vi "Pressure_Multiplexer_Server3.vi"(8 "Time per Block (s)":dbl=100.0 format="%_4f", 11 "Setup filename":string) -> (0 "DAQ Error":errorcluster, 2 "Av Sampling Rate":dbl[](array[numeric]), 3 "Time Trace":T1[](array[typedef]))   [LabVIEW 2021]
uses:
  Controls/Time_Trace_Cluster.ctl
  Controls/Setup.ctl
  Controls/Save_Data.ctl
  Camera Server/Camera enum/Camera resolution.ctl
  Globals/Meas_global.vi
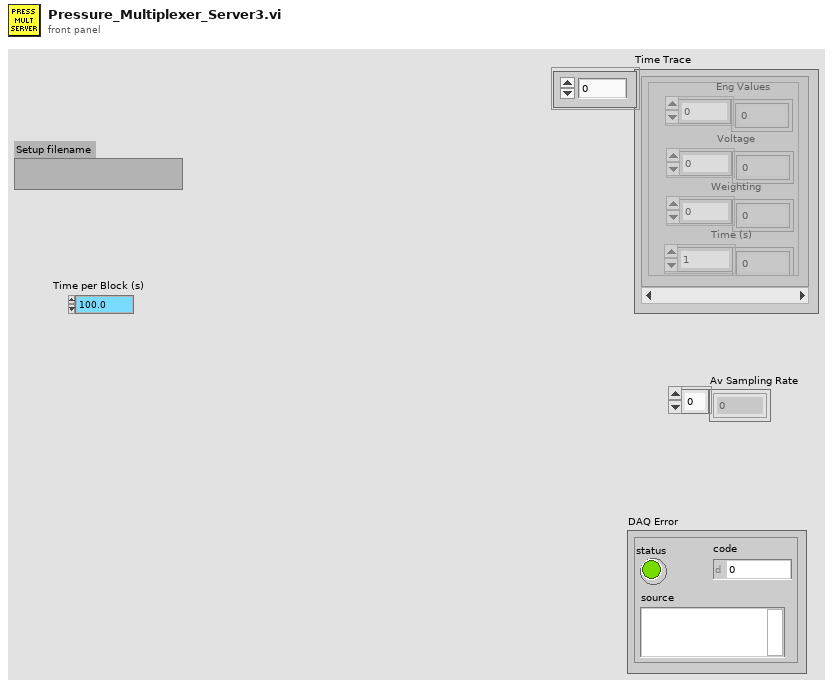
[diagram p1: front panel]
types:
  T1 = typedef "Time_Trace_Cluster.ctl" = cluster{"Weighting":dbl[], "Time (s)":dbl[], "Voltage":dbl[], "Eng Values":dbl[]}
  T2 = typedef "Save_Data.ctl" = enum16{"Save No Data", "Save Data"}
  T3 = typedef "Setup.ctl" = enum16{"Run Program", "Show Setup", "Save Current Setup", "Setup Front Panel"}
  T4 = typedef "Camera resolution.ctl" = u8
  T5 = typedef "Analysis_info_cluster.ctl" = cluster{"Colour":u32, "Inst type":T6, "Inst name":string, "Symbol":string, "Code name":string, "Extra Info":string, "Inst Array":T7, "Extra Titles":string[], "Extra Values":string[], "U":dbl, "u^2":dbl, "u^3":dbl, "u^4":dbl, "Skew_u":dbl, "Kurt_u":dbl, "Sd Error in Mean":dbl, "% u'/U":dbl, "X":dbl, "Y":dbl, "Z":dbl, "Timescale integral Estimate":dbl, "Sd Error in Variance":dbl, "Calib File":path, "Calib Constants":dbl[], "Output Position":bool, "Stats":enum16{"None", "Basic", "Full"}, "Av Sampling Rate":dbl, "Av No of Samples":dbl, "Total Meas Time (s)":dbl, "ADAM Ch Name":string, "Max value":dbl, "Min value":dbl, "Req Sample Rate Hz":dbl, "Sync Delay Time (s)":dbl, "Ch No":i16, "Device":string, "Use Latest Calib":bool, "Port":string, "Metadata Ch Names":string[], "Metadata Ch Values":string[], "Label":string}
  T6 = typedef "Inst_type.ctl" = enum16{"Raw voltage", "Raw with zero offsetting", "Propeller anemometer", "Pressure Transducer", "Pitot-static tube", "Hot wire", "Cross wire 1", "Cross wire 2", "Generic Linear", "Generic Polynomial", "Generic BackPoly", "Fast FID", "Thermocouple", "Cold wire", "Pulsed Wire", "LDA Vel", "LDA Tran time", "LDA Arr time", "Microphone"}
  T7 = typedef "Instrument_Array.ctl" = enum16{"PWA", "LDA", "Analogue"}
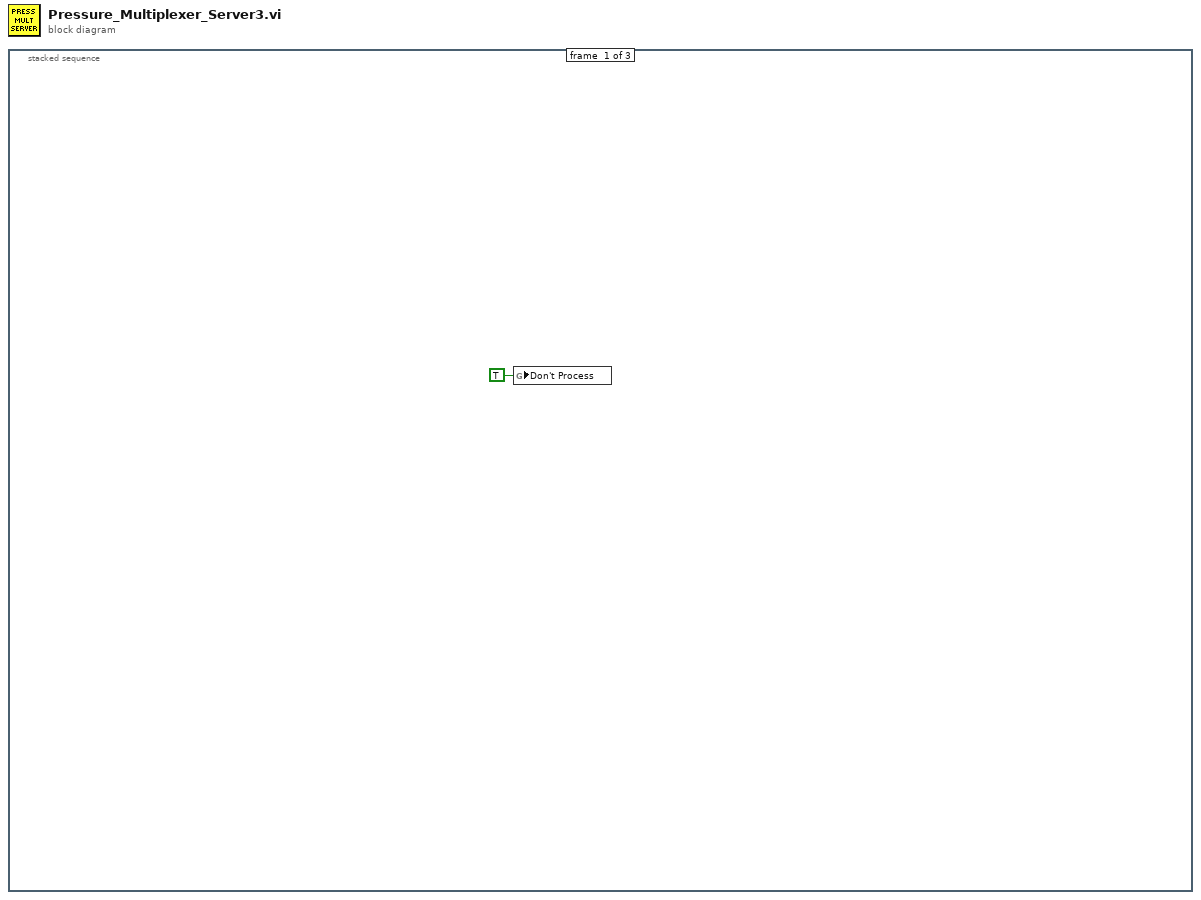
[diagram p0: block diagram]
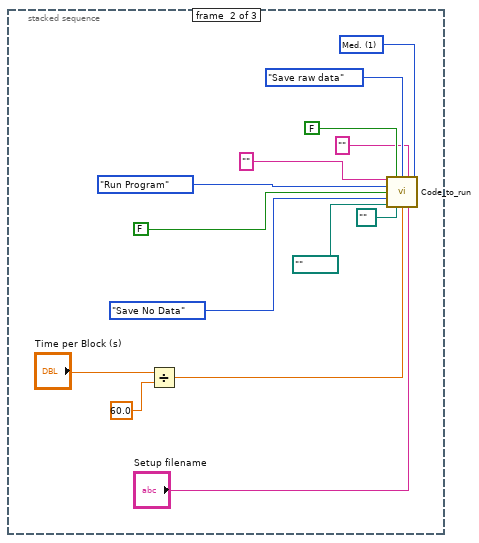
[diagram p2: hidden frame]
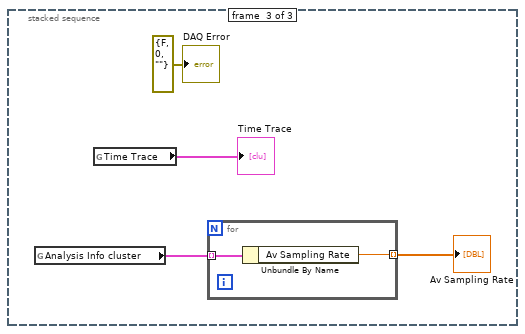
[diagram p3: hidden frame]
diagram:
  n1 = stacked-sequence {
    frame #0 {
      n2 = global write "Meas_global.vi" "Don't Process"(TRUE ("Don't Process")) -> ()
    }
    frame #1 {
      w6 = T4 1 items=["Low", "Med.", "High", "Max."] ("Camera Resolution")
      n3 = Divide(x="Time per Block (s)", y=60.0) -> (x/y=w2:dbl)
      n4 = call "Code_to_run.vi"("Extra command String"="", "Open Front Panel"=FALSE, "Raw data option"=enum16{"Save raw data", "Raw data not saved"}."Save raw data", "Current Row Comments"="", "Camera Resolution"=w6, "setup"=Setup."Run Program", "Remote control"=FALSE, "File"=Save_Data."Save No Data", "Results Filename"=path "", "Raw data file"=path "", "Averaging time (min)"=w2, "Setup filename"="Setup filename") -> ()  [unwired: 3 in, 1 out]
    }
    frame #2 {
      n5 = global read "Meas_global.vi" "Analysis Info cluster"() -> (w17:T5[])
      n6 = global read "Meas_global.vi" "Time Trace"() -> (→"Time Trace":T1[])
      n7 = for {
        tunnel: w17 -> [w21] mode=indexing
        tunnel: [w20] -> w16 mode=indexing
        n8 = Unbundle By Name(w21) -> ("Av Sampling Rate"=w20:dbl)
      }
      "Av Sampling Rate" <- w16
      "DAQ Error" <- errorcluster {"status"=FALSE, "code"=0, "source"=""} ("DAQ Error")
    }
  }
